vi "Results.vi"() -> ()   [LabVIEW 2019]
uses:
  MeasurementServer_FourProbeRawData.ctl
  MeasurementServer_ErrorOutData.ctl
  labview-grpc-measurement-server.lvlib
panel:
  out "SBC Fixture":T1[](array[typedef])=[{"Positive Voltage"=4.086739653317097e-05, "Positive Current"=0.9895248412102511, "Negative Voltage"=0.00012739710827713372, "Negative Current"=-0.988826821611341, "Impedance"=-4.37382864584101e-05, "ErrorOutData"={"ErrorCode"=-1, "ErrorMessage"="SMU HI or LO lead disconnected\n- SMU in compliance\n- SMU Fault = True\r"}}, {"Positive Voltage"=-9.910075684353424e-05, "Positive Current"=0.9823883245328239, "Negative Voltage"=0.0002639008046516521, "Negative Current"=-0.9817322721096986, "Impedance"=-0.00018481633058362254, "ErrorOutData"={"ErrorCode"=-1, "ErrorMessage"="SMU HI or LO lead disconnected\n- SMU in compliance\n- SMU Fault = True\r"}}, {"Positive Voltage"=3.8353059281555884e-05, "Positive Current"=0.9815027576624425, "Negative Voltage"=0.0001240068350202652, "Negative Current"=-0.9808838216229717, "Impedance"=-4.3647758623532466e-05, "ErrorOutData"={"ErrorCode"=-1, "ErrorMessage"="SMU HI or LO lead disconnected\n- SMU in compliance\n- SMU Fault = True\r"}}, {"Positive Voltage"=-0.00010275308356216904, "Positive Current"=0.9893423888352882, "Negative Voltage"=0.00026732713561903194, "Negative Current"=-0.9887018276515465, "Impedance"=-0.00018709400735161176, "ErrorOutData"={"ErrorCode"=-1, "ErrorMessage"="SMU HI or LO lead disconnected\n- SMU in compliance\n- SMU Fault = True\r"}}, {"Positive Voltage"=4.1695431002430516e-05, "Positive Current"=0.9812780877482301, "Negative Voltage"=0.00012506858926771908, "Negative Current"=-0.9804328544320258, "Impedance"=-4.250022593676681e-05, "ErrorOutData"={"ErrorCode"=-1, "ErrorMessage"="SMU HI or LO lead disconnected\n- SMU in compliance\n- SMU Fault = True\r"}}, {"Positive Voltage"=-9.783619149201454e-05, "Positive Current"=0.9710901411619904, "Negative Voltage"=0.00026457125211603943, "Negative Current"=-0.9703005511258349, "Impedance"=-0.00018667414294696967, "ErrorOutData"={"ErrorCode"=-1, "ErrorMessage"="SMU HI or LO lead disconnected\n- SMU in compliance\n- SMU Fault = True\r"}}, {"Positive Voltage"=3.738249995374481e-05, "Positive Current"=0.9994482162050781, "Negative Voltage"=0.00012215896581276291, "Negative Current"=-0.9989590936220989, "Impedance"=-4.242201549310266e-05, "ErrorOutData"={"ErrorCode"=-1, "ErrorMessage"="SMU HI or LO lead disconnected\n- SMU in compliance\n- SMU Fault = True\r"}}, {"Positive Voltage"=-0.0001121581250378283, "Positive Current"=0.9993179646125232, "Negative Voltage"=0.00026176653424168965, "Negative Current"=-0.9987117971097565, "Impedance"=-0.00018714669142725832, "ErrorOutData"={"ErrorCode"=-1, "ErrorMessage"="SMU HI or LO lead disconnected\n- SMU in compliance\n- SMU Fault = True\r"}}, {"Positive Voltage"=8.810060666486868e-06, "Positive Current"=0.999999516554537, "Negative Voltage"=9.118515488594028e-05, "Negative Current"=-0.9999998232497813, "Impedance"=-4.1187560705651563e-05, "ErrorOutData"={"ErrorCode"=0, "ErrorMessage"="\r"}}, {"Positive Voltage"=-0.00013435314517665922, "Positive Current"=0.9999993913728046, "Negative Voltage"=0.00023692677526758585, "Negative Current"=-0.9999995415908836, "Impedance"=-0.0001856400592644646, "ErrorOutData"={"ErrorCode"=0, "ErrorMessage"="\r"}}, {"Positive Voltage"=6.216338413542133e-06, "Positive Current"=1.0000008622581602, "Negative Voltage"=9.137275588161163e-05, "Negative Current"=-1.0000002613858447, "Impedance"=-4.2578184812673694e-05, "ErrorOutData"={"ErrorCode"=0, "ErrorMessage"="\r"}}, {"Positive Voltage"=-0.00013319308769537343, "Positive Current"=0.9999993913728046, "Negative Voltage"=0.00023524810491104786, "Negative Current"=-0.9999998545452145, "Impedance"=-0.00018422066576195294, "ErrorOutData"={"ErrorCode"=0, "ErrorMessage"="\r"}}, {"Positive Voltage"=nan, "Positive Current"=0.9999993600773714, "Negative Voltage"=nan, "Negative Current"=-0.9999997919543484, "Impedance"=nan, "ErrorOutData"={"ErrorCode"=-2, "ErrorMessage"="\rDMM HI SENSE or LO SENSE lead disconnected\n- DMM measures NaN, or \n- DMM overrange warning, or\n- DMM voltage > 50uV "}}, {"Positive Voltage"=nan, "Positive Current"=6.4894210072549e-05, "Negative Voltage"=nan, "Negative Current"=-5.418491286631952e-05, "Impedance"=nan, "ErrorOutData"={"ErrorCode"=-3, "ErrorMessage"="SMU HI or LO lead disconnected\n- SMU in compliance\n- SMU Fault = True\rDMM HI SENSE or LO SENSE lead disconnected\n- DMM measures NaN, or \n- DMM overrange warning, or\n- DMM voltage > 50uV "}}, {"Positive Voltage"=nan, "Positive Current"=0.999999234895639, "Negative Voltage"=nan, "Negative Current"=-0.9999997919543484, "Impedance"=nan, "ErrorOutData"={"ErrorCode"=-2, "ErrorMessage"="\rDMM HI SENSE or LO SENSE lead disconnected\n- DMM measures NaN, or \n- DMM overrange warning, or\n- DMM voltage > 50uV "}}, {"Positive Voltage"=nan, "Positive Current"=0.9999993913728046, "Negative Voltage"=nan, "Negative Current"=-0.9999997919543484, "Impedance"=nan, "ErrorOutData"={"ErrorCode"=-2, "ErrorMessage"="\rDMM HI SENSE or LO SENSE lead disconnected\n- DMM measures NaN, or \n- DMM overrange warning, or\n- DMM voltage > 50uV "}}, {"Positive Voltage"=nan, "Positive Current"=0.9999991723047729, "Negative Voltage"=nan, "Negative Current"=-0.999999760658915, "Impedance"=nan, "ErrorOutData"={"ErrorCode"=-2, "ErrorMessage"="\rDMM HI SENSE or LO SENSE lead disconnected\n- DMM measures NaN, or \n- DMM overrange warning, or\n- DMM voltage > 50uV "}}, {"Positive Voltage"=nan, "Positive Current"=0.999999234895639, "Negative Voltage"=nan, "Negative Current"=-0.999999760658915, "Impedance"=nan, "ErrorOutData"={"ErrorCode"=-2, "ErrorMessage"="\rDMM HI SENSE or LO SENSE lead disconnected\n- DMM measures NaN, or \n- DMM overrange warning, or\n- DMM voltage > 50uV "}}, {"Positive Voltage"=nan, "Positive Current"=0.9999992974865053, "Negative Voltage"=nan, "Negative Current"=-0.9999998232497813, "Impedance"=nan, "ErrorOutData"={"ErrorCode"=-2, "ErrorMessage"="\rDMM HI SENSE or LO SENSE lead disconnected\n- DMM measures NaN, or \n- DMM overrange warning, or\n- DMM voltage > 50uV "}}, {"Positive Voltage"=nan, "Positive Current"=0.9999993600773714, "Negative Voltage"=nan, "Negative Current"=-0.9999997919543484, "Impedance"=nan, "ErrorOutData"={"ErrorCode"=-2, "ErrorMessage"="\rDMM HI SENSE or LO SENSE lead disconnected\n- DMM measures NaN, or \n- DMM overrange warning, or\n- DMM voltage > 50uV "}}, {"Positive Voltage"=5.227425627579272e-06, "Positive Current"=0.9999990471230406, "Negative Voltage"=0.00010771239330999993, "Negative Current"=-0.9999997293634821, "Impedance"=-5.1242515189164294e-05, "ErrorOutData"={"ErrorCode"=0, "ErrorMessage"="\r"}}, {"Positive Voltage"=-0.00013780135066744496, "Positive Current"=0.9999992974865053, "Negative Voltage"=0.00025452482458244367, "Negative Current"=-0.9999997293634821, "Impedance"=-0.00019616318307304635, "ErrorOutData"={"ErrorCode"=0, "ErrorMessage"="\r"}}, {"Positive Voltage"=1.596992656295231e-05, "Positive Current"=0.9999992661910722, "Negative Voltage"=0.00010502889717128202, "Negative Current"=-0.999999760658915, "Impedance"=-4.452950697111e-05, "ErrorOutData"={"ErrorCode"=0, "ErrorMessage"="\r"}}, {"Positive Voltage"=-0.00013914746594119212, "Positive Current"=0.9999992974865053, "Negative Voltage"=0.00024127123295500423, "Negative Current"=-0.9999998232497813, "Impedance"=-0.0001902094330702244, "ErrorOutData"={"ErrorCode"=0, "ErrorMessage"="\r"}}, {"Positive Voltage"=-4.245763341031048e-06, "Positive Current"=0.9999993913728046, "Negative Voltage"=8.822880536072918e-05, "Negative Current"=-0.9999998545452145, "Impedance"=-4.6237301784238175e-05, "ErrorOutData"={"ErrorCode"=0, "ErrorMessage"="\r"}}, {"Positive Voltage"=-0.00014734412066452966, "Positive Current"=0.9999993287819383, "Negative Voltage"=0.00022868738842775972, "Negative Current"=-0.999999760658915, "Impedance"=-0.00018801584014591617, "ErrorOutData"={"ErrorCode"=0, "ErrorMessage"="\r"}}, {"Positive Voltage"=4.857765506968747e-05, "Positive Current"=0.9999992661910722, "Negative Voltage"=0.00014093281169500453, "Negative Current"=-0.9999997919543484, "Impedance"=-4.6177600058950576e-05, "ErrorOutData"={"ErrorCode"=0, "ErrorMessage"="\r"}}, {"Positive Voltage"=-0.00011304759344552028, "Positive Current"=0.9999992974865053, "Negative Voltage"=0.0002750916902080834, "Negative Current"=-0.9999997919543484, "Impedance"=-0.00019406973018278574, "ErrorOutData"={"ErrorCode"=0, "ErrorMessage"="\r"}}, {"Positive Voltage"=nan, "Positive Current"=0.9999993600773714, "Negative Voltage"=nan, "Negative Current"=-0.9999998232497813, "Impedance"=nan, "ErrorOutData"={"ErrorCode"=-2, "ErrorMessage"="\rDMM HI SENSE or LO SENSE lead disconnected\n- DMM measures NaN, or \n- DMM overrange warning, or\n- DMM voltage > 50uV "}}, {"Positive Voltage"=nan, "Positive Current"=0.9999992974865053, "Negative Voltage"=nan, "Negative Current"=-0.9999997919543484, "Impedance"=nan, "ErrorOutData"={"ErrorCode"=-2, "ErrorMessage"="\rDMM HI SENSE or LO SENSE lead disconnected\n- DMM measures NaN, or \n- DMM overrange warning, or\n- DMM voltage > 50uV "}}, {"Positive Voltage"=nan, "Positive Current"=0.9999993600773714, "Negative Voltage"=nan, "Negative Current"=-0.9999997919543484, "Impedance"=nan, "ErrorOutData"={"ErrorCode"=-2, "ErrorMessage"="\rDMM HI SENSE or LO SENSE lead disconnected\n- DMM measures NaN, or \n- DMM overrange warning, or\n- DMM voltage > 50uV "}}, {"Positive Voltage"=nan, "Positive Current"=0.9999993600773714, "Negative Voltage"=nan, "Negative Current"=-0.9999998232497813, "Impedance"=nan, "ErrorOutData"={"ErrorCode"=-2, "ErrorMessage"="\rDMM HI SENSE or LO SENSE lead disconnected\n- DMM measures NaN, or \n- DMM overrange warning, or\n- DMM voltage > 50uV "}}, {"Positive Voltage"=nan, "Positive Current"=0.9999991723047729, "Negative Voltage"=nan, "Negative Current"=-0.9999998232497813, "Impedance"=nan, "ErrorOutData"={"ErrorCode"=-2, "ErrorMessage"="\rDMM HI SENSE or LO SENSE lead disconnected\n- DMM measures NaN, or \n- DMM overrange warning, or\n- DMM voltage > 50uV "}}, {"Positive Voltage"=nan, "Positive Current"=0.9999991410093397, "Negative Voltage"=nan, "Negative Current"=-0.9999998232497813, "Impedance"=nan, "ErrorOutData"={"ErrorCode"=-2, "ErrorMessage"="\rDMM HI SENSE or LO SENSE lead disconnected\n- DMM measures NaN, or \n- DMM overrange warning, or\n- DMM voltage > 50uV "}}, {"Positive Voltage"=nan, "Positive Current"=0.9999993600773714, "Negative Voltage"=nan, "Negative Current"=-0.9999997919543484, "Impedance"=nan, "ErrorOutData"={"ErrorCode"=-2, "ErrorMessage"="\rDMM HI SENSE or LO SENSE lead disconnected\n- DMM measures NaN, or \n- DMM overrange warning, or\n- DMM voltage > 50uV "}}, {"Positive Voltage"=nan, "Positive Current"=0.9999992974865053, "Negative Voltage"=nan, "Negative Current"=-0.9999997919543484, "Impedance"=nan, "ErrorOutData"={"ErrorCode"=-2, "ErrorMessage"="\rDMM HI SENSE or LO SENSE lead disconnected\n- DMM measures NaN, or \n- DMM overrange warning, or\n- DMM voltage > 50uV "}}, {"Positive Voltage"=nan, "Positive Current"=0.9999994539636707, "Negative Voltage"=nan, "Negative Current"=-0.9999998545452145, "Impedance"=nan, "ErrorOutData"={"ErrorCode"=-2, "ErrorMessage"="\rDMM HI SENSE or LO SENSE lead disconnected\n- DMM measures NaN, or \n- DMM overrange warning, or\n- DMM voltage > 50uV "}}, {"Positive Voltage"=nan, "Positive Current"=0.9999994539636707, "Negative Voltage"=nan, "Negative Current"=-0.9999998232497813, "Impedance"=nan, "ErrorOutData"={"ErrorCode"=-2, "ErrorMessage"="\rDMM HI SENSE or LO SENSE lead disconnected\n- DMM measures NaN, or \n- DMM overrange warning, or\n- DMM voltage > 50uV "}}, {"Positive Voltage"=nan, "Positive Current"=0.9999994226682376, "Negative Voltage"=nan, "Negative Current"=-0.9999998545452145, "Impedance"=nan, "ErrorOutData"={"ErrorCode"=-2, "ErrorMessage"="\rDMM HI SENSE or LO SENSE lead disconnected\n- DMM measures NaN, or \n- DMM overrange warning, or\n- DMM voltage > 50uV "}}, {"Positive Voltage"=nan, "Positive Current"=0.9999994852591039, "Negative Voltage"=nan, "Negative Current"=-0.9999997919543484, "Impedance"=nan, "ErrorOutData"={"ErrorCode"=-2, "ErrorMessage"="\rDMM HI SENSE or LO SENSE lead disconnected\n- DMM measures NaN, or \n- DMM overrange warning, or\n- DMM voltage > 50uV "}}]
  out "Scott's Board":T1[](array[typedef])=[{"Positive Voltage"=0.0007564386469667578, "Positive Current"=0.9999993287819383, "Negative Voltage"=-0.0006195350673097383, "Negative Current"=-0.999998790500489, "Impedance"=0.0006879875040933425, "ErrorOutData"={"ErrorCode"=-2, "ErrorMessage"="\rDMM HI SENSE or LO SENSE lead disconnected\n- DMM measures NaN, or \n- DMM overrange warning, or\n- DMM voltage > 50uV "}}, {"Positive Voltage"=0.005116289340750389, "Positive Current"=1.000002708688713, "Negative Voltage"=-0.004934609355471764, "Negative Current"=-1.0000028276113588, "Impedance"=0.0050254354369517916, "ErrorOutData"={"ErrorCode"=-2, "ErrorMessage"="\rDMM HI SENSE or LO SENSE lead disconnected\n- DMM measures NaN, or \n- DMM overrange warning, or\n- DMM voltage > 50uV "}}, {"Positive Voltage"=0.0030709377367872186, "Positive Current"=0.9999996104408363, "Negative Voltage"=-0.0029474839582138124, "Negative Current"=-0.9999998232497813, "Impedance"=0.003009211699572925, "ErrorOutData"={"ErrorCode"=-2, "ErrorMessage"="\rDMM HI SENSE or LO SENSE lead disconnected\n- DMM measures NaN, or \n- DMM overrange warning, or\n- DMM voltage > 50uV "}}, {"Positive Voltage"=0.001068417768997536, "Positive Current"=0.9999993913728046, "Negative Voltage"=-0.0009405487550051928, "Negative Current"=-1.000000636931042, "Impedance"=0.0010044832477859947, "ErrorOutData"={"ErrorCode"=-2, "ErrorMessage"="\rDMM HI SENSE or LO SENSE lead disconnected\n- DMM measures NaN, or \n- DMM overrange warning, or\n- DMM voltage > 50uV "}}, {"Positive Voltage"=0.0006798617277112892, "Positive Current"=0.9999996730317025, "Negative Voltage"=-0.0005607180711459353, "Negative Current"=-0.9999998232497813, "Impedance"=0.0006202900556544055, "ErrorOutData"={"ErrorCode"=-2, "ErrorMessage"="\rDMM HI SENSE or LO SENSE lead disconnected\n- DMM measures NaN, or \n- DMM overrange warning, or\n- DMM voltage > 50uV "}}, {"Positive Voltage"=0.005099293285867178, "Positive Current"=0.9999996104408363, "Negative Voltage"=-0.004978347691753346, "Negative Current"=-0.9999999171360807, "Impedance"=0.005038821679038098, "ErrorOutData"={"ErrorCode"=-2, "ErrorMessage"="\rDMM HI SENSE or LO SENSE lead disconnected\n- DMM measures NaN, or \n- DMM overrange warning, or\n- DMM voltage > 50uV "}}, {"Positive Voltage"=0.003064458328799405, "Positive Current"=0.9999996104408363, "Negative Voltage"=-0.0029457948757943184, "Negative Current"=-0.9999999171360807, "Impedance"=0.0030051273121426167, "ErrorOutData"={"ErrorCode"=-2, "ErrorMessage"="\rDMM HI SENSE or LO SENSE lead disconnected\n- DMM measures NaN, or \n- DMM overrange warning, or\n- DMM voltage > 50uV "}}, {"Positive Voltage"=0.0010593755398858604, "Positive Current"=0.9999996104408363, "Negative Voltage"=-0.0009486398166865712, "Negative Current"=-0.9999998858406476, "Impedance"=0.0010040079311549085, "ErrorOutData"={"ErrorCode"=-2, "ErrorMessage"="\rDMM HI SENSE or LO SENSE lead disconnected\n- DMM measures NaN, or \n- DMM overrange warning, or\n- DMM voltage > 50uV "}}, {"Positive Voltage"=0.0007103462403083355, "Positive Current"=0.9999996417362693, "Negative Voltage"=-0.0006285418035758411, "Negative Current"=-0.9999998858406476, "Impedance"=0.0006694441800725301, "ErrorOutData"={"ErrorCode"=-2, "ErrorMessage"="\rDMM HI SENSE or LO SENSE lead disconnected\n- DMM measures NaN, or \n- DMM overrange warning, or\n- DMM voltage > 50uV "}}, {"Positive Voltage"=0.005072999892546784, "Positive Current"=0.9999996104408363, "Negative Voltage"=-0.004988795043902831, "Negative Current"=-0.9999999171360807, "Impedance"=0.005030898656581134, "ErrorOutData"={"ErrorCode"=-2, "ErrorMessage"="\rDMM HI SENSE or LO SENSE lead disconnected\n- DMM measures NaN, or \n- DMM overrange warning, or\n- DMM voltage > 50uV "}}, {"Positive Voltage"=0.0030662650839481816, "Positive Current"=0.9999996417362693, "Negative Voltage"=-0.0029850080581991863, "Negative Current"=-0.9999998858406476, "Impedance"=0.0030256372857641314, "ErrorOutData"={"ErrorCode"=-2, "ErrorMessage"="\rDMM HI SENSE or LO SENSE lead disconnected\n- DMM measures NaN, or \n- DMM overrange warning, or\n- DMM voltage > 50uV "}}, {"Positive Voltage"=0.0009708421061129382, "Positive Current"=0.9999996104408363, "Negative Voltage"=-0.0008834682496934806, "Negative Current"=-0.9999998858406476, "Impedance"=0.0009271554114158834, "ErrorOutData"={"ErrorCode"=-2, "ErrorMessage"="\rDMM HI SENSE or LO SENSE lead disconnected\n- DMM measures NaN, or \n- DMM overrange warning, or\n- DMM voltage > 50uV "}}, {"Positive Voltage"=nan, "Positive Current"=1.0000110332739172, "Negative Voltage"=nan, "Negative Current"=-1.0000042359058483, "Impedance"=nan, "ErrorOutData"={"ErrorCode"=-2, "ErrorMessage"="\rDMM HI SENSE or LO SENSE lead disconnected\n- DMM measures NaN, or \n- DMM overrange warning, or\n- DMM voltage > 50uV "}}, {"Positive Voltage"=nan, "Positive Current"=0.9999997356225686, "Negative Voltage"=nan, "Negative Current"=-0.9999999484315139, "Impedance"=nan, "ErrorOutData"={"ErrorCode"=-2, "ErrorMessage"="\rDMM HI SENSE or LO SENSE lead disconnected\n- DMM measures NaN, or \n- DMM overrange warning, or\n- DMM voltage > 50uV "}}, {"Positive Voltage"=nan, "Positive Current"=0.9999996104408363, "Negative Voltage"=nan, "Negative Current"=-0.9999998545452145, "Impedance"=nan, "ErrorOutData"={"ErrorCode"=-2, "ErrorMessage"="\rDMM HI SENSE or LO SENSE lead disconnected\n- DMM measures NaN, or \n- DMM overrange warning, or\n- DMM voltage > 50uV "}}, {"Positive Voltage"=nan, "Positive Current"=0.9999968877381566, "Negative Voltage"=nan, "Negative Current"=-1.0000017322712003, "Impedance"=nan, "ErrorOutData"={"ErrorCode"=-2, "ErrorMessage"="\rDMM HI SENSE or LO SENSE lead disconnected\n- DMM measures NaN, or \n- DMM overrange warning, or\n- DMM voltage > 50uV "}}, {"Positive Voltage"=nan, "Positive Current"=0.9999984525098116, "Negative Voltage"=nan, "Negative Current"=-0.9999997293634821, "Impedance"=nan, "ErrorOutData"={"ErrorCode"=-2, "ErrorMessage"="\rDMM HI SENSE or LO SENSE lead disconnected\n- DMM measures NaN, or \n- DMM overrange warning, or\n- DMM voltage > 50uV "}}, {"Positive Voltage"=nan, "Positive Current"=0.999999516554537, "Negative Voltage"=nan, "Negative Current"=-0.9999999171360807, "Impedance"=nan, "ErrorOutData"={"ErrorCode"=-2, "ErrorMessage"="\rDMM HI SENSE or LO SENSE lead disconnected\n- DMM measures NaN, or \n- DMM overrange warning, or\n- DMM voltage > 50uV "}}, {"Positive Voltage"=nan, "Positive Current"=0.99999954784997, "Negative Voltage"=nan, "Negative Current"=-0.9999998232497813, "Impedance"=nan, "ErrorOutData"={"ErrorCode"=-2, "ErrorMessage"="\rDMM HI SENSE or LO SENSE lead disconnected\n- DMM measures NaN, or \n- DMM overrange warning, or\n- DMM voltage > 50uV "}}, {"Positive Voltage"=nan, "Positive Current"=0.999999579145403, "Negative Voltage"=nan, "Negative Current"=-0.9999998232497813, "Impedance"=nan, "ErrorOutData"={"ErrorCode"=-2, "ErrorMessage"="\rDMM HI SENSE or LO SENSE lead disconnected\n- DMM measures NaN, or \n- DMM overrange warning, or\n- DMM voltage > 50uV "}}, {"Positive Voltage"=0.0007361931587577971, "Positive Current"=0.9999996417362693, "Negative Voltage"=-0.0006569520873979783, "Negative Current"=-0.9999998858406476, "Impedance"=0.0006965727876164197, "ErrorOutData"={"ErrorCode"=-2, "ErrorMessage"="\rDMM HI SENSE or LO SENSE lead disconnected\n- DMM measures NaN, or \n- DMM overrange warning, or\n- DMM voltage > 50uV "}}, {"Positive Voltage"=0.005049332720968932, "Positive Current"=0.9999996104408363, "Negative Voltage"=-0.004967798618501576, "Negative Current"=-0.9999998545452145, "Impedance"=0.005008567009561862, "ErrorOutData"={"ErrorCode"=-2, "ErrorMessage"="\rDMM HI SENSE or LO SENSE lead disconnected\n- DMM measures NaN, or \n- DMM overrange warning, or\n- DMM voltage > 50uV "}}, {"Positive Voltage"=0.00304491083857335, "Positive Current"=0.9999996104408363, "Negative Voltage"=-0.0029551384843021678, "Negative Current"=-0.9999999171360807, "Impedance"=0.0030000253700783763, "ErrorOutData"={"ErrorCode"=-2, "ErrorMessage"="\rDMM HI SENSE or LO SENSE lead disconnected\n- DMM measures NaN, or \n- DMM overrange warning, or\n- DMM voltage > 50uV "}}, {"Positive Voltage"=0.0010119912692798285, "Positive Current"=0.9999996104408363, "Negative Voltage"=-0.000942197798896207, "Negative Current"=-0.9999998858406476, "Impedance"=0.000977094780178384, "ErrorOutData"={"ErrorCode"=-2, "ErrorMessage"="\rDMM HI SENSE or LO SENSE lead disconnected\n- DMM measures NaN, or \n- DMM overrange warning, or\n- DMM voltage > 50uV "}}, {"Positive Voltage"=0.0006921431321562702, "Positive Current"=0.9999997043271356, "Negative Voltage"=-0.0006354869842074939, "Negative Current"=-0.9999999171360807, "Impedance"=0.0006638151838211144, "ErrorOutData"={"ErrorCode"=-2, "ErrorMessage"="\rDMM HI SENSE or LO SENSE lead disconnected\n- DMM measures NaN, or \n- DMM overrange warning, or\n- DMM voltage > 50uV "}}, {"Positive Voltage"=0.005032954530404898, "Positive Current"=0.9999996104408363, "Negative Voltage"=-0.004977520186973587, "Negative Current"=-0.9999998858406476, "Impedance"=0.005005238619304928, "ErrorOutData"={"ErrorCode"=-2, "ErrorMessage"="\rDMM HI SENSE or LO SENSE lead disconnected\n- DMM measures NaN, or \n- DMM overrange warning, or\n- DMM voltage > 50uV "}}, {"Positive Voltage"=0.003093091101621005, "Positive Current"=0.9999996104408363, "Negative Voltage"=-0.002927110030067358, "Negative Current"=-0.9999998545452145, "Impedance"=0.003010101371067292, "ErrorOutData"={"ErrorCode"=-2, "ErrorMessage"="\rDMM HI SENSE or LO SENSE lead disconnected\n- DMM measures NaN, or \n- DMM overrange warning, or\n- DMM voltage > 50uV "}}, {"Positive Voltage"=0.0010682629335981378, "Positive Current"=0.9999996417362693, "Negative Voltage"=-0.0009396090540731372, "Negative Current"=-0.9999998858406476, "Impedance"=0.0010039362309769624, "ErrorOutData"={"ErrorCode"=-2, "ErrorMessage"="\rDMM HI SENSE or LO SENSE lead disconnected\n- DMM measures NaN, or \n- DMM overrange warning, or\n- DMM voltage > 50uV "}}, {"Positive Voltage"=nan, "Positive Current"=0.999999579145403, "Negative Voltage"=nan, "Negative Current"=-0.9999998545452145, "Impedance"=nan, "ErrorOutData"={"ErrorCode"=-2, "ErrorMessage"="\rDMM HI SENSE or LO SENSE lead disconnected\n- DMM measures NaN, or \n- DMM overrange warning, or\n- DMM voltage > 50uV "}}, {"Positive Voltage"=nan, "Positive Current"=0.99999954784997, "Negative Voltage"=nan, "Negative Current"=-0.9999998232497813, "Impedance"=nan, "ErrorOutData"={"ErrorCode"=-2, "ErrorMessage"="\rDMM HI SENSE or LO SENSE lead disconnected\n- DMM measures NaN, or \n- DMM overrange warning, or\n- DMM voltage > 50uV "}}, {"Positive Voltage"=nan, "Positive Current"=0.999999579145403, "Negative Voltage"=nan, "Negative Current"=-0.9999999171360807, "Impedance"=nan, "ErrorOutData"={"ErrorCode"=-2, "ErrorMessage"="\rDMM HI SENSE or LO SENSE lead disconnected\n- DMM measures NaN, or \n- DMM overrange warning, or\n- DMM voltage > 50uV "}}, {"Positive Voltage"=nan, "Positive Current"=0.999999579145403, "Negative Voltage"=nan, "Negative Current"=-0.9999998858406476, "Impedance"=nan, "ErrorOutData"={"ErrorCode"=-2, "ErrorMessage"="\rDMM HI SENSE or LO SENSE lead disconnected\n- DMM measures NaN, or \n- DMM overrange warning, or\n- DMM voltage > 50uV "}}, {"Positive Voltage"=nan, "Positive Current"=0.999999579145403, "Negative Voltage"=nan, "Negative Current"=-0.9999998858406476, "Impedance"=nan, "ErrorOutData"={"ErrorCode"=-2, "ErrorMessage"="\rDMM HI SENSE or LO SENSE lead disconnected\n- DMM measures NaN, or \n- DMM overrange warning, or\n- DMM voltage > 50uV "}}, {"Positive Voltage"=nan, "Positive Current"=0.999999579145403, "Negative Voltage"=nan, "Negative Current"=-0.9999999171360807, "Impedance"=nan, "ErrorOutData"={"ErrorCode"=-2, "ErrorMessage"="\rDMM HI SENSE or LO SENSE lead disconnected\n- DMM measures NaN, or \n- DMM overrange warning, or\n- DMM voltage > 50uV "}}, {"Positive Voltage"=nan, "Positive Current"=0.9999996104408363, "Negative Voltage"=nan, "Negative Current"=-0.9999998545452145, "Impedance"=nan, "ErrorOutData"={"ErrorCode"=-2, "ErrorMessage"="\rDMM HI SENSE or LO SENSE lead disconnected\n- DMM measures NaN, or \n- DMM overrange warning, or\n- DMM voltage > 50uV "}}, {"Positive Voltage"=nan, "Positive Current"=0.99999954784997, "Negative Voltage"=nan, "Negative Current"=-0.9999998545452145, "Impedance"=nan, "ErrorOutData"={"ErrorCode"=-2, "ErrorMessage"="\rDMM HI SENSE or LO SENSE lead disconnected\n- DMM measures NaN, or \n- DMM overrange warning, or\n- DMM voltage > 50uV "}}, {"Positive Voltage"=nan, "Positive Current"=0.999999579145403, "Negative Voltage"=nan, "Negative Current"=-0.9999999171360807, "Impedance"=nan, "ErrorOutData"={"ErrorCode"=-2, "ErrorMessage"="\rDMM HI SENSE or LO SENSE lead disconnected\n- DMM measures NaN, or \n- DMM overrange warning, or\n- DMM voltage > 50uV "}}, {"Positive Voltage"=nan, "Positive Current"=0.999999579145403, "Negative Voltage"=nan, "Negative Current"=-0.9999998858406476, "Impedance"=nan, "ErrorOutData"={"ErrorCode"=-2, "ErrorMessage"="\rDMM HI SENSE or LO SENSE lead disconnected\n- DMM measures NaN, or \n- DMM overrange warning, or\n- DMM voltage > 50uV "}}, {"Positive Voltage"=nan, "Positive Current"=0.999999579145403, "Negative Voltage"=nan, "Negative Current"=-0.9999998858406476, "Impedance"=nan, "ErrorOutData"={"ErrorCode"=-2, "ErrorMessage"="\rDMM HI SENSE or LO SENSE lead disconnected\n- DMM measures NaN, or \n- DMM overrange warning, or\n- DMM voltage > 50uV "}}, {"Positive Voltage"=nan, "Positive Current"=0.999999579145403, "Negative Voltage"=nan, "Negative Current"=-0.9999998232497813, "Impedance"=nan, "ErrorOutData"={"ErrorCode"=-2, "ErrorMessage"="\rDMM HI SENSE or LO SENSE lead disconnected\n- DMM measures NaN, or \n- DMM overrange warning, or\n- DMM voltage > 50uV "}}]
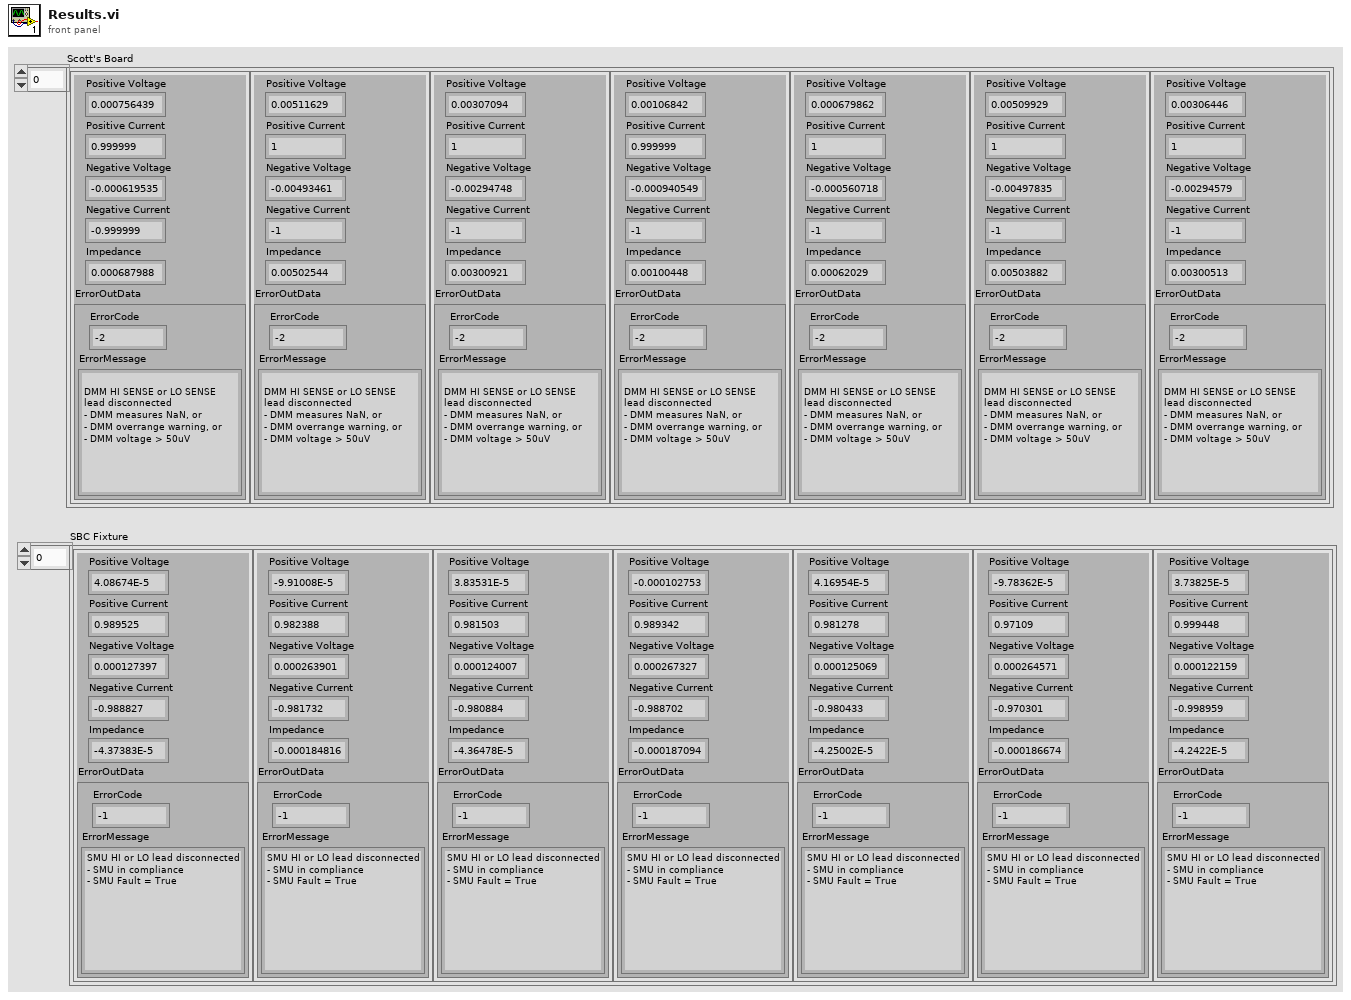
[diagram p1: front panel]
types:
  T1 = typedef "labview-grpc-measurement-server.lvlib/MeasurementServer_FourProbeRawData.ctl" = cluster{"Positive Voltage":dbl, "Positive Current":dbl, "Negative Voltage":dbl, "Negative Current":dbl, "Impedance":dbl, "ErrorOutData":T2}
  T2 = typedef "labview-grpc-measurement-server.lvlib/MeasurementServer_ErrorOutData.ctl" = cluster{"ErrorCode":i32, "ErrorMessage":string}
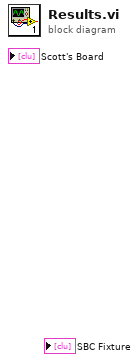
[diagram p0: block diagram]
diagram:
